vi "Read Cosine.vi"(8 "error in (no error)":errorcluster, 11 "NI-Scope Lock-in Driver in":refnum<class "NI-Scope Lock-in Driver.lvclass">) -> (0 "error out":errorcluster, 2 "Cosine":dbl[](array[numeric]), 3 "NI-Scope Lock-in Driver out":refnum<class "NI-Scope Lock-in Driver.lvclass">)   [LabVIEW 2016, in "NI-Scope Lock-in Driver.lvclass"]
uses:
  NI-Scope Lock-in Driver.lvclass
  NI-Scope Lock-in Driver.lvclass/NI-Scope Lock-in Driver.ctl
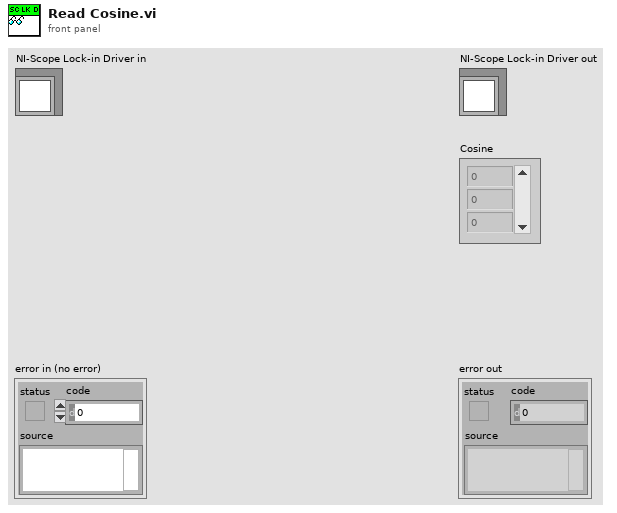
[diagram p1: front panel]
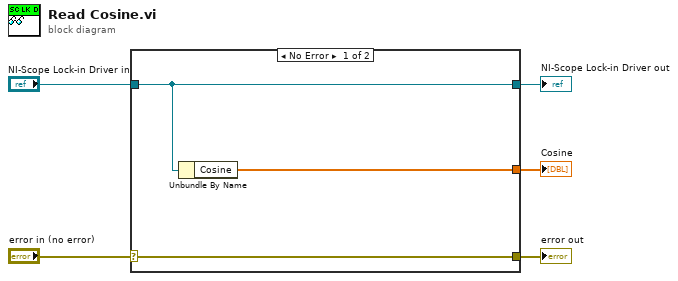
[diagram p0: block diagram]
diagram:
  n1 = case shown="No Error" "error in (no error)" {
    selector: "error in (no error)" -> [w8 w9]
    tunnel: [w8 w9] -> w4
    tunnel: [w7 w10] -> w2
    tunnel: "NI-Scope Lock-in Driver in" -> [w7 w10]
    tunnel: [w6 _] -> w1
    frame No Error {
      n2 = Unbundle By Name(w7) -> ("Cosine"=w6:dbl[])
    }
    frame Error {
    }
  }
  "error out" <- w4
  "NI-Scope Lock-in Driver out" <- w2
  "Cosine" <- w1
